vi "data to booleans.vi"(9 "specifications":T1[](array[typedef]), 10 "allocation":bool[](array[boolean]), 11 "data table":T3) -> (2 "registers":bool[](array[boolean]), 3 "allocation":T3)   [LabVIEW 2013, in "Modbus Slave runtime.lvclass"]
uses:
  Modbus Slave runtime.lvclass
  <vilib>/NI/Tag Bus/table/data table.ctl
  data mapping elements.ctl
  <vilib>/NI/Tag Bus/tag/Data Type.ctl
  <vilib>/NI/Tag Bus/table/data polymorphs/read one/read Double.vi
  <vilib>/NI/Tag Bus/table/data polymorphs/read one/read Single.vi
  <vilib>/NI/Tag Bus/table/data polymorphs/read one/read I64.vi
  <vilib>/NI/Tag Bus/table/data polymorphs/read one/read U64.vi
  <vilib>/NI/Tag Bus/table/data polymorphs/read one/read I32.vi
  <vilib>/NI/Tag Bus/table/data polymorphs/read one/read U32.vi
  <vilib>/NI/Tag Bus/table/data polymorphs/read one/read I16.vi
  <vilib>/NI/Tag Bus/table/data polymorphs/read one/read U16.vi
  <vilib>/NI/Tag Bus/table/data polymorphs/read one/read I8.vi
  <vilib>/NI/Tag Bus/table/data polymorphs/read one/read U8.vi
  <vilib>/NI/Tag Bus/table/data polymorphs/read one/read Boolean.vi
  <vilib>/NI/Tag Bus/table/data table.lvlib
  <vilib>/NI/Tag Bus/tag/tag descriptor.lvclass
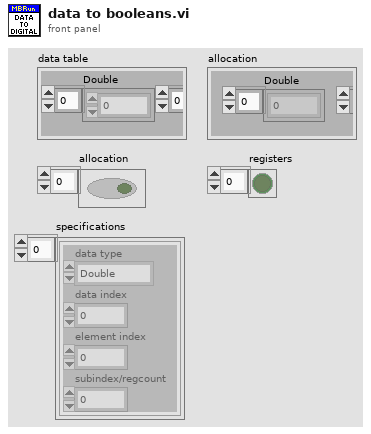
[diagram p1: front panel]
types:
  T1 = typedef "Modbus Slave runtime.lvclass/data mapping elements.ctl" = cluster{"data type":T2, "data index":i32, "element index":i32, "subindex/regcount":i32}
  T2 = typedef "tag bus.lvlib/tag descriptor.lvclass/Data Type.ctl" = enum16{"Double", "Single", "I64", "I32", "I16", "I8", "U64", "U32", "U16", "U8", "Boolean", "String", "Array of Double", "Array of Single", "Array of I64", "Array of I32", "Array of I16", "Array of I8", "Array of U64", "Array of U32", "Array of U16", "Array of U8", "Array of Boolean", "Array of String"}
  T3 = typedef "tag bus.lvlib/data table.lvlib/data table.ctl" = cluster{"Double":dbl[], "Single":sgl[], "I64":i64[], "I32":i32[], "I16":i16[], "I8":i8[], "U64":u64[], "U32":u32[], "U16":u16[], "U8":u8[], "Boolean":bool[], "String":string[], "Array of Double":cluster{"DBL Array":dbl[]}[], "Array of Single":cluster{"SGL Array":sgl[]}[], "Array of I64":cluster{"I64 Array":i64[]}[], "Array of I32":cluster{"I32 Array":i32[]}[], "Array of I16":cluster{"I16 Array":i16[]}[], "Array of I8":cluster{"I8 Array":i8[]}[], "Array of U64":cluster{"U64 Array":u64[]}[], "Array of U32":cluster{"U32 Array":u32[]}[], "Array of U16":cluster{"U16 Array":u16[]}[], "Array of U8":cluster{"U8 Array":u8[]}[], "Array of Boolean":cluster{"Boolean Array":bool[]}[], "Array of String":cluster{"String Array":string[]}[]}
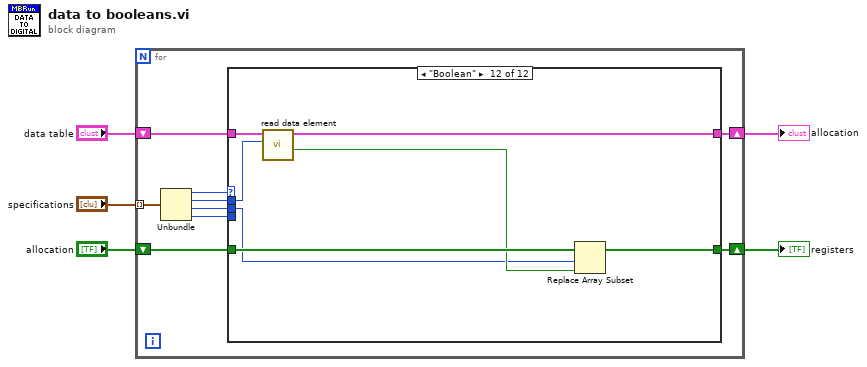
[diagram p0: block diagram]
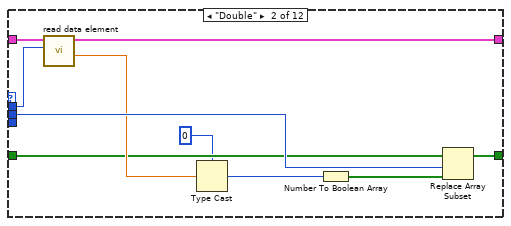
[diagram p3: hidden frame]
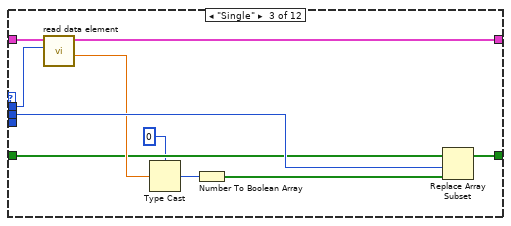
[diagram p4: hidden frame]
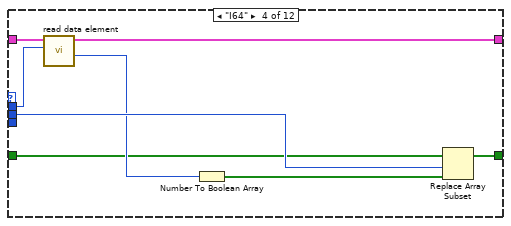
[diagram p5: hidden frame]
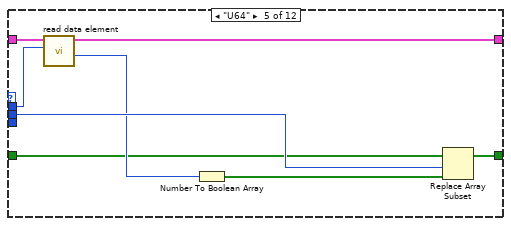
[diagram p6: hidden frame]
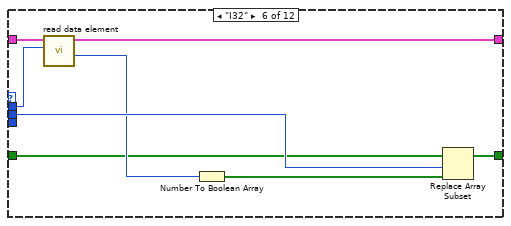
[diagram p7: hidden frame]
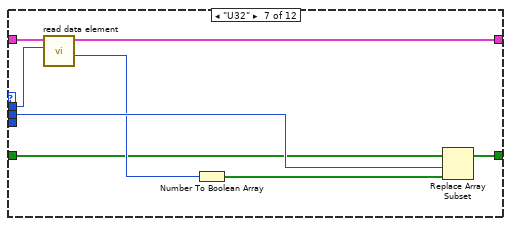
[diagram p8: hidden frame]
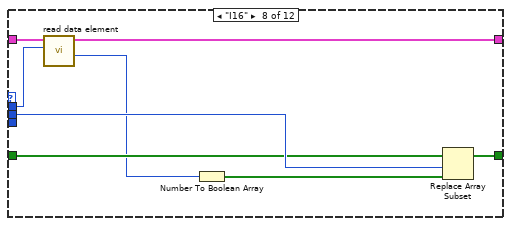
[diagram p9: hidden frame]
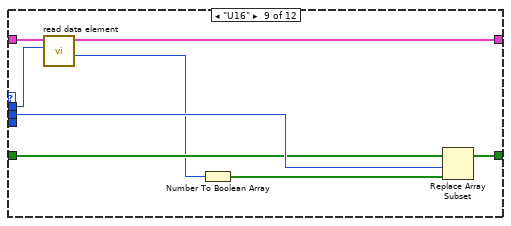
[diagram p10: hidden frame]
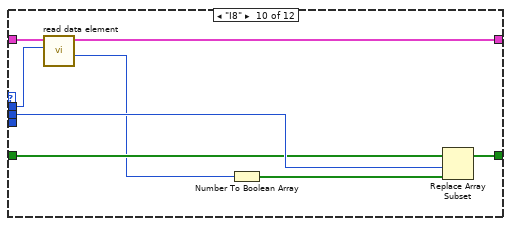
[diagram p11: hidden frame]
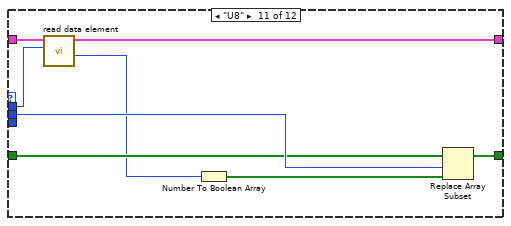
[diagram p12: hidden frame]
diagram:
  n1 = for {
    shift-right: [w11] -> w4
    shift-left: "data table" -> [w12]
    tunnel: "specifications" -> [w14] mode=indexing
    shift-right: [w7] -> w1
    shift-left: "allocation" -> [w10]
    n2 = Unbundle(w14) -> ("data type"=w13:T2, "data index"=w9:i32, "element index"=w6:i32, "subindex/regcount"=w8:i32)
    n3 = case shown="\"Boolean\"" w13 {
      tunnel: w12 -> [w16 w26 w36 w44 w52 w60 w68 w76 w84 w92 w100 w107]
      tunnel: [w16 w25 w35 w43 w51 w59 w67 w75 w83 w91 w99 w106] -> w11
      tunnel: w6 -> [_ w22 w32 w40 w48 w56 w64 w72 w80 w88 w96 w101]
      tunnel: w10 -> [w15 w20 w30 w38 w46 w54 w62 w71 w79 w87 w95 w103]
      tunnel: w9 -> [_ w24 w34 w42 w50 w58 w66 w74 w82 w90 w98 w105]
      tunnel: w8 -> [_ _ _ _ _ _ _ _ _ _ _ _]
      tunnel: [w15 w23 w33 w41 w49 w57 w65 w73 w81 w89 w97 w104] -> w7
      frame Default {
      }
      frame "Double" {
        n4 = call-poly <vilib>:"read data element.vi"("index"=w24, "data table in"=w26) -> ("value"=w21:dbl, "data table out"=w25:T3)  [unwired: 8 in]
        n5 = Type Cast(type=u64 0, x=w21) -> (*(type *) &x=w19:u64)
        n6 = Number To Boolean Array(number=w19) -> (Boolean array=w17:bool[])
        n7 = Replace Array Subset(array=w20, new element=w17, index=w22) -> (w23:bool[])
      }
      frame "Single" {
        n8 = call-poly <vilib>:"read data element.vi"("index"=w34, "data table in"=w36) -> ("value"=w31:sgl, "data table out"=w35:T3)  [unwired: 8 in]
        n9 = Type Cast(type=u32 0, x=w31) -> (*(type *) &x=w28:u32)
        n10 = Number To Boolean Array(number=w28) -> (Boolean array=w29:bool[])
        n11 = Replace Array Subset(array=w30, new element=w29, index=w32) -> (w33:bool[])
      }
      frame "I64" {
        n12 = call-poly <vilib>:"read data element.vi"("index"=w42, "data table in"=w44) -> ("value"=w39:i64, "data table out"=w43:T3)  [unwired: 8 in]
        n13 = Number To Boolean Array(number=w39) -> (Boolean array=w37:bool[])
        n14 = Replace Array Subset(array=w38, new element=w37, index=w40) -> (w41:bool[])
      }
      frame "U64" {
        n15 = call-poly <vilib>:"read data element.vi"("index"=w50, "data table in"=w52) -> ("value"=w47:u64, "data table out"=w51:T3)  [unwired: 8 in]
        n16 = Number To Boolean Array(number=w47) -> (Boolean array=w45:bool[])
        n17 = Replace Array Subset(array=w46, new element=w45, index=w48) -> (w49:bool[])
      }
      frame "I32" {
        n18 = call-poly <vilib>:"read data element.vi"("index"=w58, "data table in"=w60) -> ("value"=w55:i32, "data table out"=w59:T3)  [unwired: 8 in]
        n19 = Number To Boolean Array(number=w55) -> (Boolean array=w53:bool[])
        n20 = Replace Array Subset(array=w54, new element=w53, index=w56) -> (w57:bool[])
      }
      frame "U32" {
        n21 = call-poly <vilib>:"read data element.vi"("index"=w66, "data table in"=w68) -> ("value"=w63:u32, "data table out"=w67:T3)  [unwired: 8 in]
        n22 = Number To Boolean Array(number=w63) -> (Boolean array=w61:bool[])
        n23 = Replace Array Subset(array=w62, new element=w61, index=w64) -> (w65:bool[])
      }
      frame "I16" {
        n24 = call-poly <vilib>:"read data element.vi"("index"=w74, "data table in"=w76) -> ("value"=w70:i16, "data table out"=w75:T3)  [unwired: 8 in]
        n25 = Number To Boolean Array(number=w70) -> (Boolean array=w69:bool[])
        n26 = Replace Array Subset(array=w71, new element=w69, index=w72) -> (w73:bool[])
      }
      frame "U16" {
        n27 = call-poly <vilib>:"read data element.vi"("index"=w82, "data table in"=w84) -> ("value"=w78:u16, "data table out"=w83:T3)  [unwired: 8 in]
        n28 = Number To Boolean Array(number=w78) -> (Boolean array=w77:bool[])
        n29 = Replace Array Subset(array=w79, new element=w77, index=w80) -> (w81:bool[])
      }
      frame "I8" {
        n30 = call-poly <vilib>:"read data element.vi"("index"=w90, "data table in"=w92) -> ("value"=w86:i8, "data table out"=w91:T3)  [unwired: 8 in]
        n31 = Number To Boolean Array(number=w86) -> (Boolean array=w85:bool[])
        n32 = Replace Array Subset(array=w87, new element=w85, index=w88) -> (w89:bool[])
      }
      frame "U8" {
        n33 = call-poly <vilib>:"read data element.vi"("index"=w98, "data table in"=w100) -> ("value"=w94:u8, "data table out"=w99:T3)  [unwired: 8 in]
        n34 = Number To Boolean Array(number=w94) -> (Boolean array=w93:bool[])
        n35 = Replace Array Subset(array=w95, new element=w93, index=w96) -> (w97:bool[])
      }
      frame "Boolean" {
        n36 = call-poly <vilib>:"read data element.vi"("index"=w105, "data table in"=w107) -> ("value"=w102:bool, "data table out"=w106:T3)  [unwired: 8 in]
        n37 = Replace Array Subset(array=w103, new element=w102, index=w101) -> (w104:bool[])
      }
    }
  }
  "allocation" <- w4
  "registers" <- w1
